vi "RP convert raw data.vi"(7 "Max Volts":sgl[](array[numeric])=[20.0, 1.0], 8 "Error In":errorcluster, 9 "Signal bits":i32=14, 10 "Format":T1=enum."Digitizer", 11 "data stream":string) -> (0 "Error Out":errorcluster, 1 "element":u32, 2 "phase out":u32[](array[numeric]), 3 "data out":sgl[][](array[numeric]))   [LabVIEW 2015]
uses:
  Mode.ctl
  RP ADC to Volts 1D.vi
  RP 32 ADC to Volts 1D.vi
  RP ADC to Volts 2D.vi
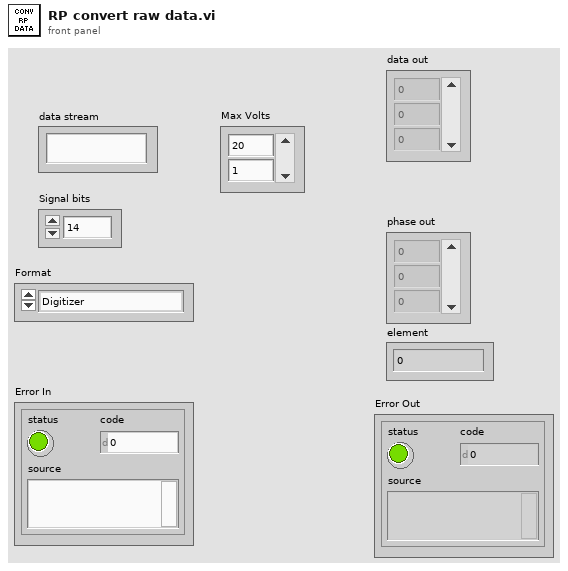
[diagram p1: front panel]
types:
  T1 = typedef "Mode.ctl" = enum16{"Filter", "Lockin test", "Snapshot test", "Digitizer", "Current-Voltage"}
  T2 = enum16{"big-endian, network order", "native, host order", "little-endian"}
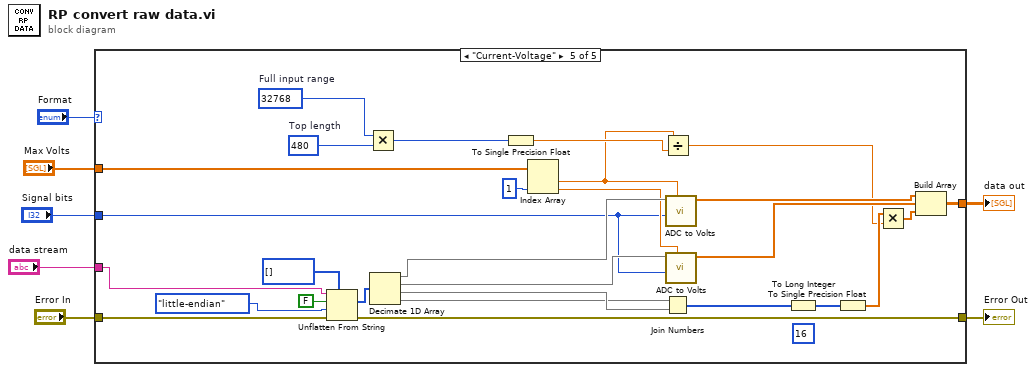
[diagram p0: block diagram]
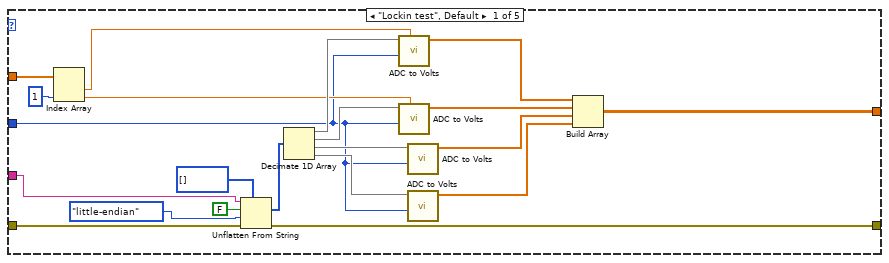
[diagram p2: hidden frame]
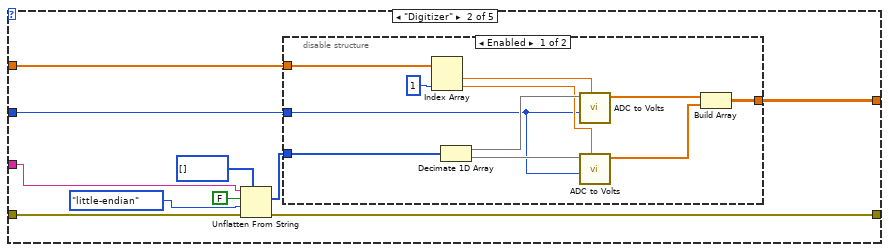
[diagram p3: hidden frame]
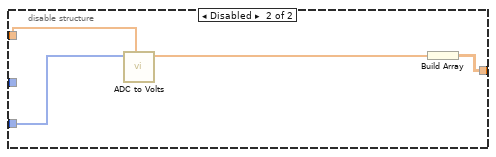
[diagram p4: hidden frame]
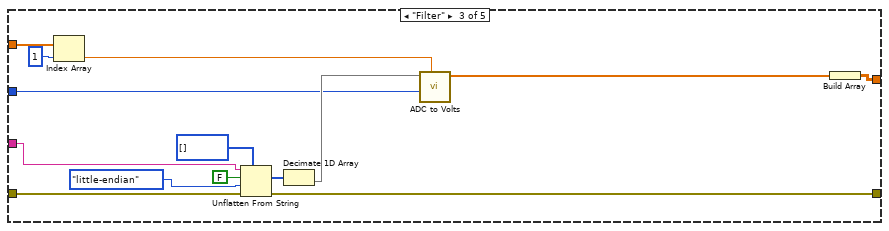
[diagram p5: hidden frame]
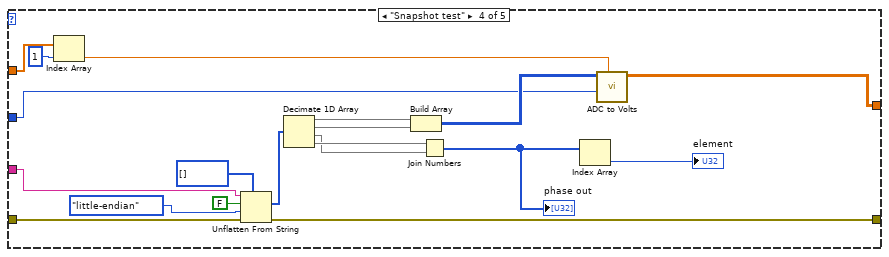
[diagram p6: hidden frame]
diagram:
  n1 = case shown="\"Current-Voltage\"" "Format" {
    tunnel: [w28 w31 w67 w81 w102] -> w5
    tunnel: "Max Volts" -> [w19 w32 w64 w80 w114]
    tunnel: "data stream" -> [w13 w36 w61 w76 w110]
    tunnel: "Error In" -> [w14 w35 w60 w74 w108]
    tunnel: [w12 w30 w57 w73 w107] -> w2
    tunnel: "Signal bits" -> [w8 w29 w54 w68 w91]
    frame "Lockin test", Default {
      n2 = Index Array(array=w19, index #2=1 ("index")) -> (element #1=w11:sgl, element #2=w10:sgl)  [unwired: 1 in]
      n3 = Unflatten From String(type=i16[] [], binary string=w13, data includes array or string size? (T)=FALSE, byte order (0:big-endian, network order)=T2."little-endian", error in (no error)=w14) -> (value=w15:i16[], error out=w12:errorcluster)  [unwired: 1 out]
      n4 = Decimate 1D Array(w15) -> (w27:i16[], w25:i16[], w23:i16[], w22:i16[])
      n5 = call-poly "ADC to Volts.vi"("Max Volts"=w11, "Signal bits"=w8, "ADC data"=w27) -> ("Volts"=w26:sgl[])  [unwired: 8 in]
      n6 = call-poly "ADC to Volts.vi"("Max Volts"=w10, "Signal bits"=w8, "ADC data"=w25) -> ("Volts"=w24:sgl[])  [unwired: 8 in]
      n7 = call-poly "ADC to Volts.vi"("Signal bits"=w8, "ADC data"=w23) -> ("Volts"=w20:sgl[])  [unwired: 9 in]
      n8 = call-poly "ADC to Volts.vi"("Signal bits"=w8, "ADC data"=w22) -> ("Volts"=w21:sgl[])  [unwired: 9 in]
      n9 = Build Array(w26, w24, w20, w21) -> (w28:sgl[][])
    }
    frame "Digitizer" {
      n10 = Unflatten From String(type=i16[] [], binary string=w36, data includes array or string size? (T)=FALSE, byte order (0:big-endian, network order)=T2."little-endian", error in (no error)=w35) -> (value=w33:i16[], error out=w30:errorcluster)  [unwired: 1 out]
      n11 = disable-structure shown="Enabled" {
        disable-tunnel: [w44 w50] -> w31
        disable-tunnel: w33 -> [w49 w52]
        disable-tunnel: w32 -> [w42 w53]
        disable-tunnel: w29 -> [w39 _]
        frame Enabled {
          n12 = Index Array(array=w42, index #2=1 ("index")) -> (element #1=w40:sgl, element #2=w41:sgl)  [unwired: 1 in]
          n13 = Decimate 1D Array(w49) -> (w48:i16[], w47:i16[])
          n14 = call-poly "ADC to Volts.vi"("Max Volts"=w40, "Signal bits"=w39, "ADC data"=w48) -> ("Volts"=w46:sgl[])  [unwired: 8 in]
          n15 = call-poly "ADC to Volts.vi"("Max Volts"=w41, "Signal bits"=w39, "ADC data"=w47) -> ("Volts"=w45:sgl[])  [unwired: 8 in]
          n16 = Build Array(w46, w45) -> (w44:sgl[][])
        }
        frame Disabled {
          n17 = call-poly "ADC to Volts.vi"("Max Volts"=w53, "ADC data"=w52) -> ("Volts"=w51:sgl[])  [unwired: 9 in]
          n18 = Build Array(w51) -> (w50:sgl[][])
        }
      }
    }
    frame "Filter" {
      n19 = Index Array(array=w64, index=1) -> (element=w56:sgl)
      n20 = Unflatten From String(type=i32[] [], binary string=w61, data includes array or string size? (T)=FALSE, byte order (0:big-endian, network order)=T2."little-endian", error in (no error)=w60) -> (value=w58:i32[], error out=w57:errorcluster)  [unwired: 1 out]
      n21 = Decimate 1D Array(w58) -> (w66:i32[])  [unwired: 1 out]
      n22 = call-poly "ADC to Volts.vi"("Max Volts"=w56, "Signal bits"=w54, "ADC data"=w66) -> ("Volts"=w65:sgl[])  [unwired: 8 in]
      n23 = Build Array(w65) -> (w67:sgl[][])
    }
    frame "Snapshot test" {
      n24 = Index Array(array=w80, index=1) -> (element=w72:sgl)
      n25 = Unflatten From String(type=i16[] [], binary string=w76, data includes array or string size? (T)=FALSE, byte order (0:big-endian, network order)=T2."little-endian", error in (no error)=w74) -> (value=w75:i16[], error out=w73:errorcluster)  [unwired: 1 out]
      n26 = Decimate 1D Array(w75) -> (w86:i16[], w85:i16[], w83:i16[], w84:i16[])
      n27 = Build Array(w86, w85) -> (w82:i16[][])
      n28 = Join Numbers(hi=w84, lo=w83) -> ((hi.lo)=w70:u32[])
      "phase out" <- w70
      n29 = Index Array(array=w70) -> (element=→"element":u32)  [unwired: 1 in]
      n30 = call-poly "ADC to Volts.vi"("Max Volts"=w72, "Signal bits"=w68, "ADC data"=w82) -> ("Volts"=w81:sgl[][])  [unwired: 8 in]
    }
    frame "Current-Voltage" {
      (unwired) 16 ("Signal bits")
      w105 = 480  # Top length
      w106 = 32768  # Full input range
      n31 = Unflatten From String(type=i16[] [], binary string=w110, data includes array or string size? (T)=FALSE, byte order (0:big-endian, network order)=T2."little-endian", error in (no error)=w108) -> (value=w109:i16[], error out=w107:errorcluster)  [unwired: 1 out]
      n32 = Multiply(x=w106, y=w105) -> (x*y=w103:i32)
      n33 = Decimate 1D Array(w109) -> (w97:i16[], w96:i16[], w100:i16[], w99:i16[])
      n34 = To Single Precision Float(number=w103) -> (single precision float=w88:sgl)
      n35 = Index Array(array=w114, index #2=1 ("index")) -> (element #1=w87:sgl, element #2=w92:sgl)  [unwired: 1 in]
      n36 = Divide(x=w87, y=w88) -> (x/y=w89:sgl)
      n37 = Join Numbers(hi=w99, lo=w100) -> ((hi.lo)=w98:u32[])
      n38 = call-poly "ADC to Volts.vi"("Max Volts"=w87, "Signal bits"=w91, "ADC data"=w97) -> ("Volts"=w95:sgl[])  [unwired: 8 in]
      n39 = call-poly "ADC to Volts.vi"("Max Volts"=w92, "Signal bits"=w91, "ADC data"=w96) -> ("Volts"=w94:sgl[])  [unwired: 8 in]
      n40 = To Long Integer(number=w98) -> (32bit integer=w90:i32[])
      n41 = To Single Precision Float(number=w90) -> (single precision float=w104:sgl[])
      n42 = Multiply(x=w104, y=w89) -> (x*y=w101:sgl[])
      n43 = Build Array(w95, w94, w101) -> (w102:sgl[][])
    }
  }
  "Error Out" <- w2
  "data out" <- w5
